vi "WriteValue_DBL.vi"(9 "value":dbl, 11 "reference":refnum<vi>) -> ()   [LabVIEW 2012]
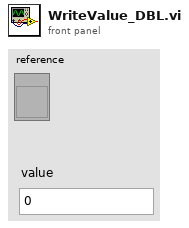
[diagram p1: front panel]
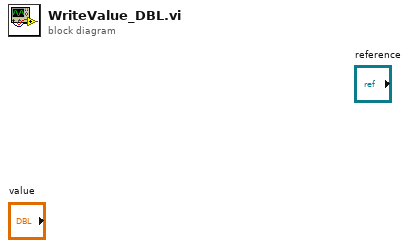
[diagram p0: block diagram]
diagram:
